vi "SETMIXTUREdll.vi"(8 "error in (no error)":errorcluster, 11 "hmixnme":string) -> (0 "error out":errorcluster, 1 "hmixnme_length":i32, 2 "ierr":i32, 3 "z":dbl[](array[numeric]))   [LabVIEW 2016]
doc: "subroutine SETMIXTUREdll(hmixnme, z, ierr, hmixnme_length)\n\nCall the SETMIX routine for a predefined mixture without the need to pass hfmix, hrf, ncc, hf, or herr. It is not\nnecessary to declare the length of hmixnme as 255 bytes long. A path can be included if needed. The extension\n“.mix” is not required. If it is necessary to set the reference state, call subroutine FLAGS first. The composition\nof the mixture will be returned in the z array. If ierr comes back non-zero, call the ERRMSG routine to obtain\nit.\n\nExamples:\ncall SETMIXTURE ('AIR.MIX',z,ierr) ! load the air mixture from the AIR.MIX file\ncall SETMIXTURE ('C:/REFPROP/MIXTURES/AIR.MIX',z,ierr) read the AIR.MIX file from the C:/REFPROP/MIXTURES directory\ncall SETMIXTURE ('R410A.MIX',z,ierr) ! load the R410A mixture, the composition will be returned on a mole percent basis in the z array.\ncall SETMIXTURE ('R410A',z,ierr) ! works the same as above for predefined refrigerant mixtures that start with R4 or R5.\n\nINPUTS:\nhmixnme -- String of any character length containing the mixture file name\n\nOUTPUTS:\nz -- Composition array (mole fractions)\nierr -- Error flag. 0 Successful (Values are identical to SETMIX)\nhmixnme_length -- length of variable hmixnme (default: 10000)"
uses:
  REFPROP.DLL
panel:
  # "REFPROP-SETMIXTUREdll.vi"
  # "void  SETMIXTUREdll(CStr hmixnme, double *z, int32_t *ierr, int32_t hmixnme_length);"
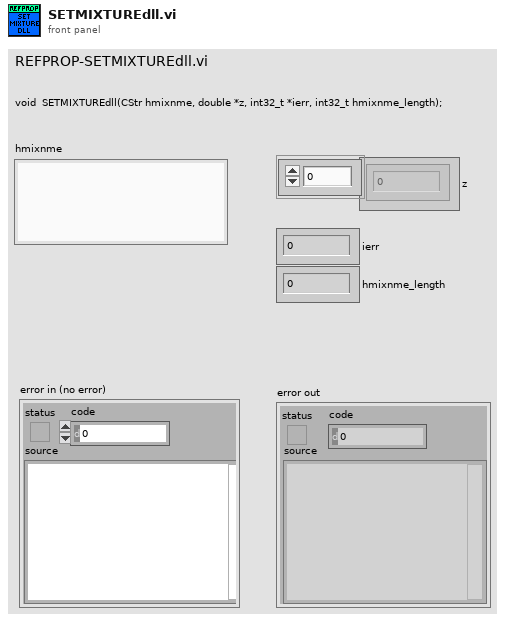
[diagram p1: front panel]
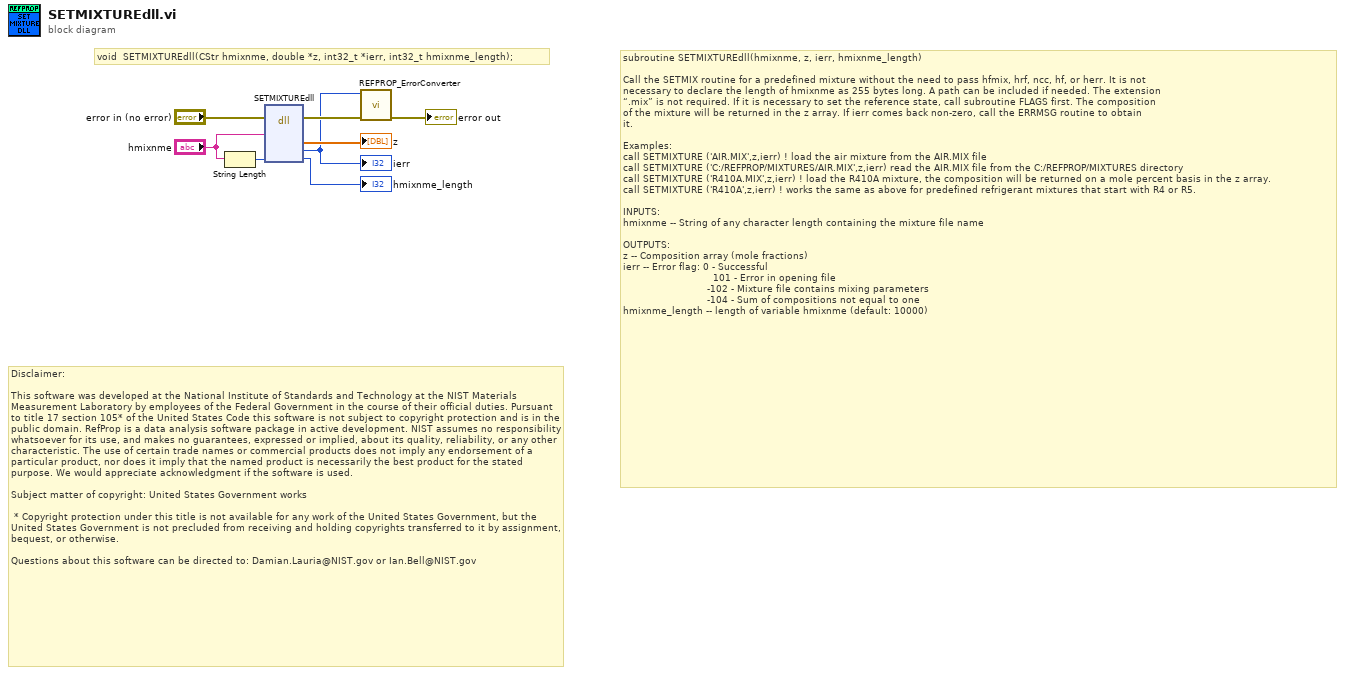
[diagram p0: block diagram]
diagram:
  # "void  SETMIXTUREdll(CStr hmixnme, double *z, int32_t *ierr, int32_t hmixnme_length);"
  # "subroutine SETMIXTUREdll(hmixnme, z, ierr, hmixnme_length)\n\nCall the SETMIX routine for a predefined mixture without the need to pass hfmix, hrf, ncc, hf, or herr. It is not\nnecessary to declare the length of hmixnme as 255 bytes long. A path can be included if needed. The extension\n“.mix” is not required. If it is necessary to set the reference state, call subroutine FLAGS first. The composition\nof the mixture will be returned in the z array. If ierr comes back non-zero, call the ERRMSG routine to obtain\nit.\n\nExamples:\ncall SETMIXTURE ('AIR.MIX',z,ierr) ! load the air mixture from the AIR.MIX file\ncall SETMIXTURE ('C:/REFPROP/MIXTURES/AIR.MIX',z,ierr) read the AIR.MIX file from the C:/REFPROP/MIXTURES directory\ncall SETMIXTURE ('R410A.MIX',z,ierr) ! load the R410A mixture, the composition will be returned on a mole percent basis in the z array.\ncall SETMIXTURE ('R410A',z,ierr) ! works the same as above for predefined refrigerant mixtures that start with R4 or R5.\n\nINPUTS:\nhmixnme -- String of any character length containing the mixture file name\n\nOUTPUTS:\nz -- Composition array (mole fractions)\nierr -- Error flag: 0 - Successful \n                              101 - Error in opening file \n                            -102 - Mixture file contains mixing parameters \n                            -104 - Sum of compositions not equal to one\nhmixnme_length -- length of variable hmixnme (default: 10000)"
  # "Disclaimer:\n\nThis software was developed at the National Institute of Standards and Technology at the NIST Materials Measurement Laboratory by employees of the Federal Government in the course of their official duties. Pursuant to title 17 section 105* of the United States Code this software is not subject to copyright protection and is in the public domain. RefProp is a data analysis software package in active development. NIST assumes no responsibility whatsoever for its use, and makes no guarantees, expressed or implied, about its quality, reliability, or any other characteristic. The use of certain trade names or commercial products does not imply any endorsement of a particular product, nor does it imply that the named product is necessarily the best product for the stated purpose. We would appreciate acknowledgment if the software is used.\n \nSubject matter of copyright: United States Government works\n  \n * Copyright protection under this title is not available for any work of the United States Government, but the United States Government is not precluded from receiving and holding copyrights transferred to it by assignment, bequest, or otherwise.\n\nQuestions about this software can be directed to: Damian.Lauria@NIST.gov or Ian.Bell@NIST.gov"
  n1 = String Length(string="hmixnme") -> (length=w2:i32)
  n2 = dll-call lib="S:/009 - Testing/02 - Performance Testing/REFPROP/REFPROP.*" fn="SETMIXTUREdll"(error in="error in (no error)", "hmixnme"="hmixnme", "hmixnme_length"=w2) -> (error out=w8:errorcluster, "z"=→"z":dbl[], "ierr"=w4:i32, "hmixnme_length"=→"hmixnme_length":i32)  [unwired: 6 in, 1 out]
  "ierr" <- w4
  n3 = call "REFPROP_ErrorConverter.vi"("error in (no error)"=w8, "Error Code"=w4) -> ("error out"=→"error out":errorcluster)  [unwired: 9 in]
